vi "Find RetVal Components.vi"(8 "Error In":errorcluster, 11 "Proto Method VI":refnum<vi>) -> (0 "Error Out":errorcluster, 1 "Indicator":refnum<vi>, 2 "Data Buffer":refnum<vi>, 3 "Proto Method VI Dup":refnum<vi>, 4 "Wire":refnum<vi>)   [LabVIEW 2013, in "Abstract Param Writer.lvclass"]
doc: "Copyright (c) 2016 Sze Howe Koh\n\nThis Source Code Form is subject to the terms of the Mozilla Public License, v. 2.0. If a copy of the MPL was not distributed with this file, You can obtain one at http://mozilla.org/MPL/2.0/."
uses:
  Abstract Param Writer.lvclass
  <vilib>/Utility/traverseref.llb/TRef TravTarget.ctl
  <vilib>/Utility/traverseref.llb/VI Scripting - Traverse.lvlib
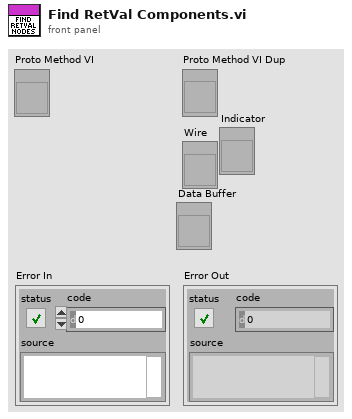
[diagram p1: front panel]
types:
  T1 = typedef "TRef TravTarget.ctl" = enum16{"FP", "BD", "Other"}
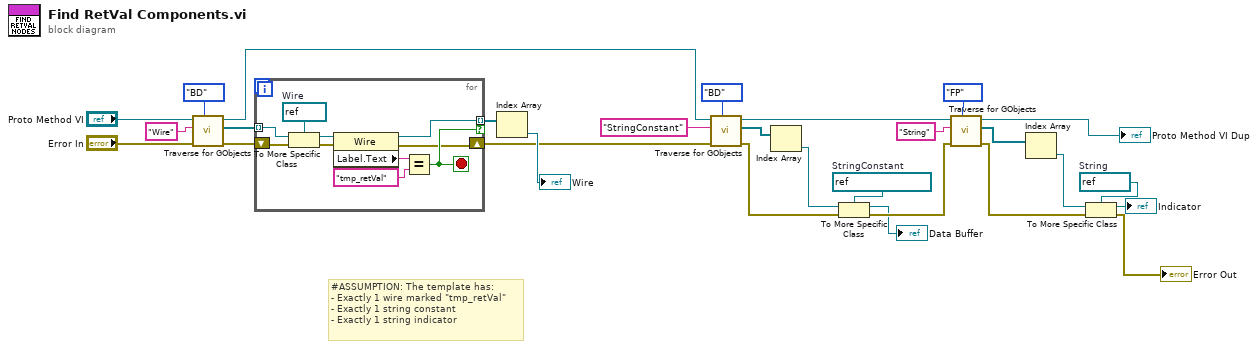
[diagram p0: block diagram]
diagram:
  w4 = refnum<vi> refnum  # String
  w12 = refnum<vi> refnum  # StringConstant
  # "#ASSUMPTION: The template has:\n- Exactly 1 wire marked \"tmp_retVal\"\n- Exactly 1 string constant\n- Exactly 1 string indicator"
  n1 = call <vilib>:"Traverse for GObjects.vi"("Traverse Target"=TRef_TravTarget."BD", "error in (no error)"="Error In", "Class Name"="Wire", "VI Refnum"="Proto Method VI") -> ("error out"=w23:errorcluster, "References"=w25:refnum<vi>[], "dup VI Refnum"=w18:refnum<vi>)  [unwired: 4 in, 1 out]
  n2 = for {
    tunnel: w25 -> [w38] mode=indexing
    tunnel: [w33] -> w24 mode=indexing if=w32
    shift-right: [w29] -> w17
    shift-left: w23 -> [w30]
    stop <- w32 stop-if-true
    w37 = refnum<vi> refnum  # Wire
    n3 = To More Specific Class(target class=w37, reference=w38, error in=w30) -> (specific class reference=w36:refnum<vi>, error out=w31:errorcluster)
    n4 = property class="Wire"(reference=w36, error in=w31) -> (reference out=w33:refnum<vi>, error out=w29:errorcluster, "Label.Text"=w35:string)
    n5 = Equal?(x=w35, y="tmp_retVal") -> (x = y?=w32:bool)
  }
  n6 = Index Array(array=w24) -> (element=→"Wire":refnum<vi>)  [unwired: 1 in]
  n7 = call <vilib>:"Traverse for GObjects.vi"("Traverse Target"=TRef_TravTarget."BD", "error in (no error)"=w17, "Class Name"="StringConstant", "VI Refnum"=w18) -> ("error out"=w10:errorcluster, "References"=w16:refnum<vi>[], "dup VI Refnum"=w13:refnum<vi>)  [unwired: 4 in, 1 out]
  n8 = Index Array(array=w16) -> (element=w11:refnum<vi>)  [unwired: 1 in]
  n9 = To More Specific Class(target class=w12, reference=w11, error in=w10) -> (specific class reference=→"Data Buffer":refnum<vi>, error out=w9:errorcluster)
  n10 = call <vilib>:"Traverse for GObjects.vi"("Traverse Target"=TRef_TravTarget."FP", "error in (no error)"=w9, "Class Name"="String", "VI Refnum"=w13) -> ("error out"=w7:errorcluster, "References"=w6:refnum<vi>[], "dup VI Refnum"=→"Proto Method VI Dup":refnum<vi>)  [unwired: 4 in, 1 out]
  n11 = Index Array(array=w6) -> (element=w5:refnum<vi>)  [unwired: 1 in]
  n12 = To More Specific Class(target class=w4, reference=w5, error in=w7) -> (specific class reference=→"Indicator":refnum<vi>, error out=→"Error Out":errorcluster)
